vi "判断查询是否包括今日.vi"(11 "日期时间条件":cluster{"年":i32, "月":i32, "周":i32, "日":i32}) -> (2 "条件语句":T1, 3 "查询类型":T2)   [LabVIEW 2013, in "数据库操作.lvclass"]
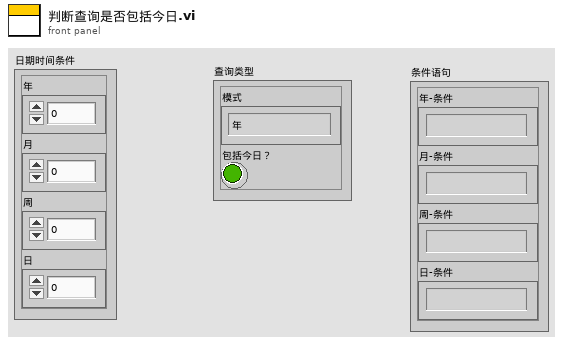
[diagram p1: front panel]
types:
  T1 = cluster{"年-条件":string, "月-条件":string, "周-条件":string, "日-条件":string}
  T2 = cluster{"模式":enum16{"年", "月", "周", "日"}, "包括今日？":bool}
  T3 = typedef "LVDateTimeRec.ctl" = cluster{"秒数的小数部分":dbl, "秒":i32, "分":i32, "时":i32, "日":i32, "月":i32, "年":i32, "天数（周）":i32, "天数（年）":i32, "DST":i32}
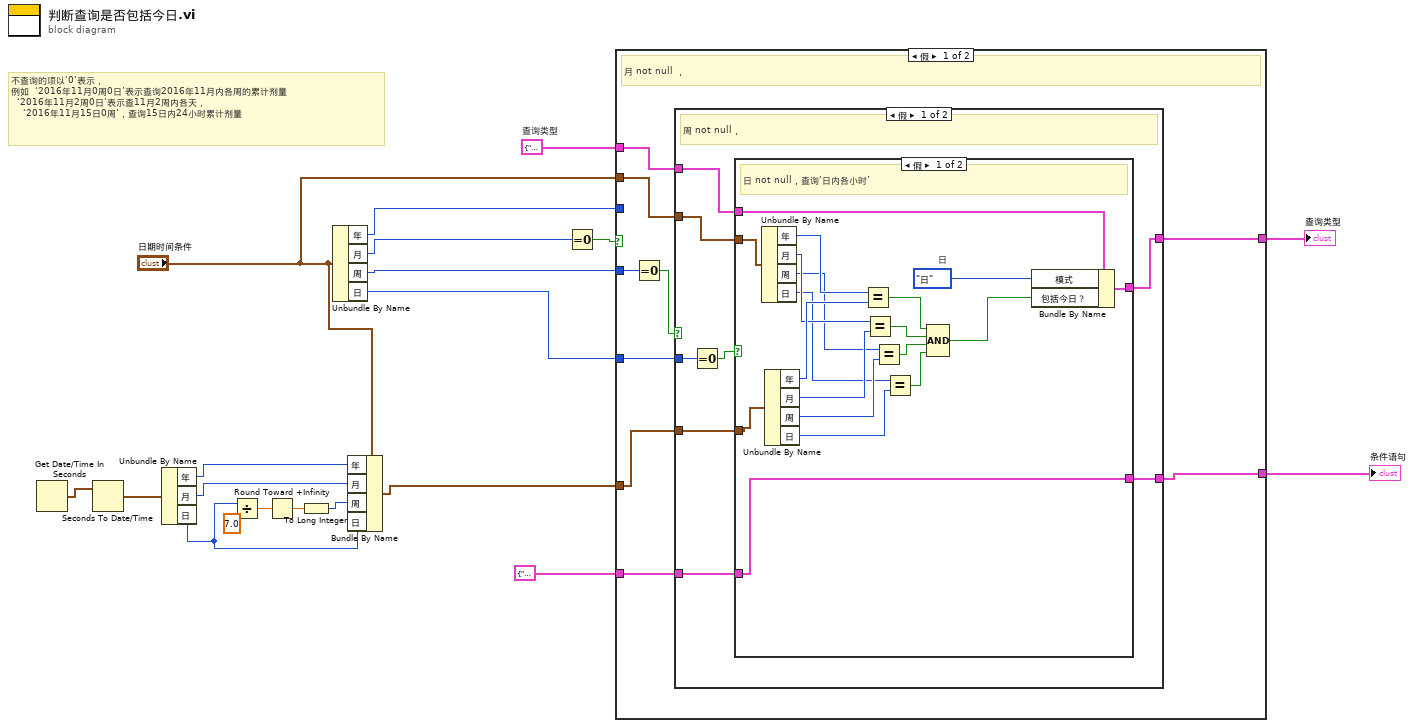
[diagram p0: block diagram]
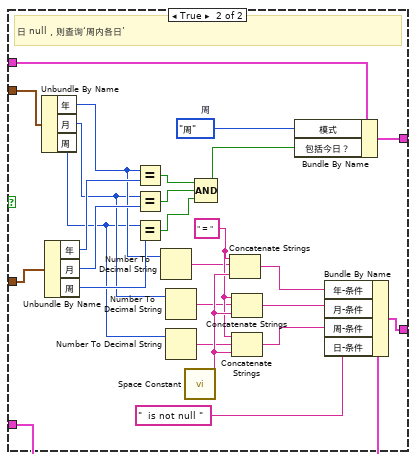
[diagram p2: hidden frame]
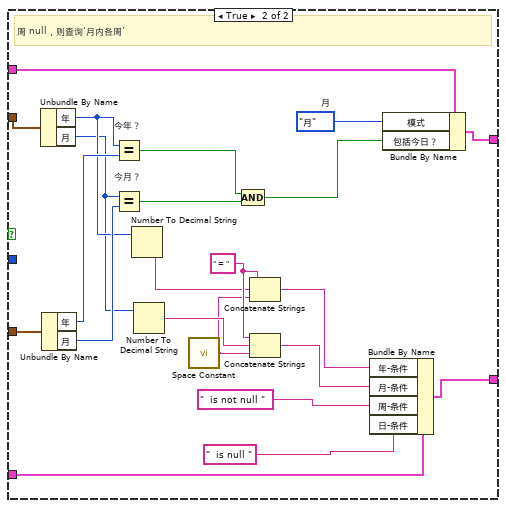
[diagram p3: hidden frame]
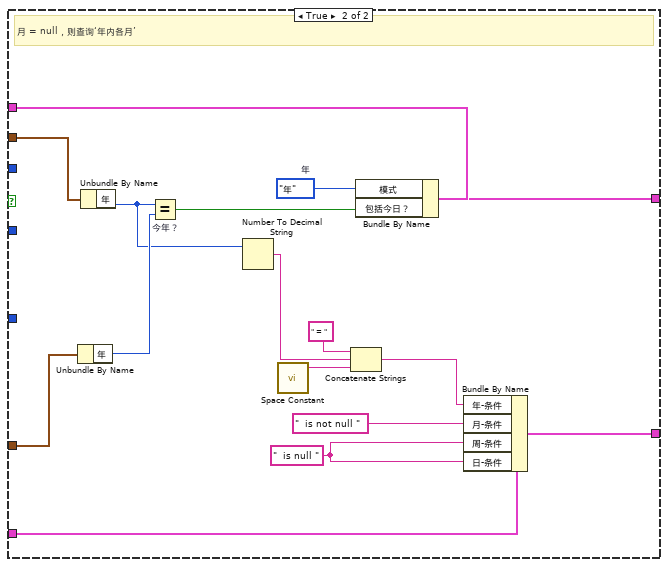
[diagram p4: hidden frame]
diagram:
  w5 = T2 {"模式"=enum."年", "包括今日？"=FALSE}  # 查询类型
  # "不查询的项以‘0’表示，\n例如  ‘2016年11月0周0日’表示查询2016年11月内各周的累计剂量\n  ‘2016年11月2周0日’表示查11月2周内各天，\n    ‘2016年11月15日0周’，查询15日内24小时累计剂量"
  n1 = Get Date/Time In Seconds() -> (seconds since 1Jan1904=w20:timestamp)
  n2 = Seconds To Date/Time(time stamp (now)=w20) -> (date time rec=w19:T3)  [unwired: 1 in]
  n3 = Unbundle By Name(w19) -> ("年"=w11:i32, "月"=w10:i32, "日"=w8:i32)
  n4 = Divide(x=w8, y=7.0) -> (x/y=w17:dbl)
  n5 = Round Toward +Infinity(x=w17) -> (ceil(x): smallest int >= x=w16:dbl)
  n6 = To Long Integer(number=w16) -> (32bit integer=w9:i32)
  n7 = Unbundle By Name("日期时间条件") -> ("年"=w6:i32, "月"=w15:i32, "周"=w13:i32, "日"=w12:i32)
  n8 = Bundle By Name(cluster="日期时间条件", "年"=w11, "月"=w10, "周"=w9, "日"=w8) -> (w7:cluster{"年":i32, "月":i32, "周":i32, "日":i32})
  n9 = Equal To 0?(x=w15) -> (x = 0?=w14:bool)
  n10 = case shown="假" w14 {
    tunnel: w13 -> [w29 _]
    tunnel: w12 -> [w27 _]
    tunnel: w7 -> [w26 w120]
    tunnel: w6 -> [_ _]
    tunnel: w5 -> [w23 w118]
    tunnel: [w24 w115] -> w3
    tunnel: "日期时间条件" -> [w25 w114]
    tunnel: T1 {"年-条件"="", "月-条件"="", "周-条件"="", "日-条件"=""} ("条件语句") -> [w22 w113]
    tunnel: [w21 w106] -> w1
    frame False {
      # "月 not null ，"
      n11 = Equal To 0?(x=w29) -> (x = 0?=w28:bool)
      n12 = case shown="假" w28 {
        tunnel: w27 -> [w37 _]
        tunnel: w26 -> [w34 w104]
        tunnel: w25 -> [w35 w103]
        tunnel: [w32 w96] -> w24
        tunnel: w23 -> [w33 w95]
        tunnel: w22 -> [w31 w94]
        tunnel: [w30 w83] -> w21
        frame False {
          # "周 not null，"
          n13 = Equal To 0?(x=w37) -> (x = 0?=w36:bool)
          n14 = case shown="假" w36 {
            tunnel: w35 -> [w44 w80]
            tunnel: w34 -> [w43 w79]
            tunnel: w33 -> [w55 w81]
            tunnel: [w54 w71] -> w32
            tunnel: w31 -> [w38 w70]
            tunnel: [w38 w57] -> w30
            frame False {
              w56 = enum16{"年", "月", "周", "日"}."日"  # 日
              # "日 not null，查询‘日内各小时’"
              n15 = Unbundle By Name(w44) -> ("年"=w42:i32, "月"=w41:i32, "周"=w40:i32, "日"=w39:i32)
              n16 = Unbundle By Name(w43) -> ("年"=w53:i32, "月"=w52:i32, "周"=w51:i32, "日"=w50:i32)
              n17 = Equal?(x=w42, y=w53) -> (x = y?=w49:bool)
              n18 = Equal?(x=w41, y=w52) -> (x = y?=w48:bool)
              n19 = Equal?(x=w40, y=w51) -> (x = y?=w47:bool)
              n20 = Equal?(x=w39, y=w50) -> (x = y?=w46:bool)
              n21 = Compound Arithmetic op=AND(w49, w48, w47, w46) -> (w45:bool)
              n22 = Bundle By Name(cluster=w55, "模式"=w56, "包括今日？"=w45) -> (w54:T2)
            }
            frame True {
              w64 = " = " ("字符串")
              w82 = enum16{"年", "月", "周", "日"}."周"  # 周
              # "日 null，则查询‘周内各日’"
              n23 = Unbundle By Name(w80) -> ("年"=w68:i32, "月"=w67:i32, "周"=w66:i32)
              n24 = Unbundle By Name(w79) -> ("年"=w78:i32, "月"=w77:i32, "周"=w76:i32)
              n25 = Equal?(x=w68, y=w78) -> (x = y?=w75:bool)
              n26 = Equal?(x=w67, y=w77) -> (x = y?=w74:bool)
              n27 = Equal?(x=w66, y=w76) -> (x = y?=w73:bool)
              n28 = Number To Decimal String(number=w68) -> (decimal integer string=w63:string)  [unwired: 1 in]
              n29 = Number To Decimal String(number=w67) -> (decimal integer string=w62:string)  [unwired: 1 in]
              n30 = Number To Decimal String(number=w66) -> (decimal integer string=w61:string)  [unwired: 1 in]
              n31 = call <vilib>:"Space Constant.vi"() -> ("String"=w65:string)
              n32 = Compound Arithmetic op=AND(w75, w74, w73) -> (w72:bool)
              n33 = Concatenate Strings(w64, w63, w65) -> (w59:string)
              n34 = Concatenate Strings(w64, w62, w65) -> (w60:string)
              n35 = Concatenate Strings(w64, w61, w65) -> (w58:string)
              n36 = Bundle By Name(cluster=w81, "模式"=w82, "包括今日？"=w72) -> (w71:T2)
              n37 = Bundle By Name(cluster=w70, "年-条件"=w59, "月-条件"=w60, "周-条件"=w58, "日-条件"="  is not null " ("月-条件")) -> (w57:T1)
            }
          }
        }
        frame True {
          w91 = " = " ("字符串")
          w98 = enum16{"年", "月", "周", "日"}."月"  # 月
          # "周 null，则查询‘月内各周’"
          n38 = Unbundle By Name(w103) -> ("年"=w93:i32, "月"=w92:i32)
          n39 = Unbundle By Name(w104) -> ("年"=w102:i32, "月"=w101:i32)
          n40 = Equal? "今年？"(x=w93, y=w102) -> (x = y?=w100:bool)
          n41 = Equal? "今月？"(x=w92, y=w101) -> (x = y?=w99:bool)
          n42 = Number To Decimal String(number=w93) -> (decimal integer string=w90:string)  [unwired: 1 in]
          n43 = Number To Decimal String(number=w92) -> (decimal integer string=w89:string)  [unwired: 1 in]
          n44 = call <vilib>:"Space Constant.vi"() -> ("String"=w87:string)
          n45 = Compound Arithmetic op=AND(w100, w99) -> (w97:bool)
          n46 = Concatenate Strings(w91, w90, w87) -> (w88:string)
          n47 = Concatenate Strings(w91, w89, w87) -> (w86:string)
          n48 = Bundle By Name(cluster=w94, "年-条件"=w88, "月-条件"=w86, "周-条件"="  is not null " ("月-条件"), "日-条件"="  is null " ("周-条件")) -> (w83:T1)
          n49 = Bundle By Name(cluster=w95, "模式"=w98, "包括今日？"=w97) -> (w96:T2)
        }
      }
    }
    frame True {
      w107 = "  is null " ("周-条件")
      w116 = enum16{"年", "月", "周", "日"}."年"  # 年
      # "月 = null，则查询‘年内各月’"
      n50 = Unbundle By Name(w120) -> ("年"=w119:i32)
      n51 = Unbundle By Name(w114) -> ("年"=w111:i32)
      n52 = Equal? "今年？"(x=w111, y=w119) -> (x = y?=w117:bool)
      n53 = Number To Decimal String(number=w111) -> (decimal integer string=w109:string)  [unwired: 1 in]
      n54 = call <vilib>:"Space Constant.vi"() -> ("String"=w105:string)
      n55 = Concatenate Strings(" = " ("字符串"), w109, w105) -> (w108:string)
      n56 = Bundle By Name(cluster=w118, "模式"=w116, "包括今日？"=w117) -> (w115:T2)
      n57 = Bundle By Name(cluster=w113, "年-条件"=w108, "月-条件"="  is not null ", "周-条件"=w107, "日-条件"=w107) -> (w106:T1)
    }
  }
  "查询类型" <- w3
  "条件语句" <- w1
